vi "agent_sign.vi"() -> ()   [LabVIEW 2017]
doc: "Illustrates how to sign data using an ssh2-agent."
uses:
  libssh2/libssh2_init_default.vi
  libssh2/libssh2_session_init_ex.vi
  libssh2/libssh2.lvlib
panel:
  out "signature":string
  in  "data":string="Hello, World!"
  out "error out":errorcluster
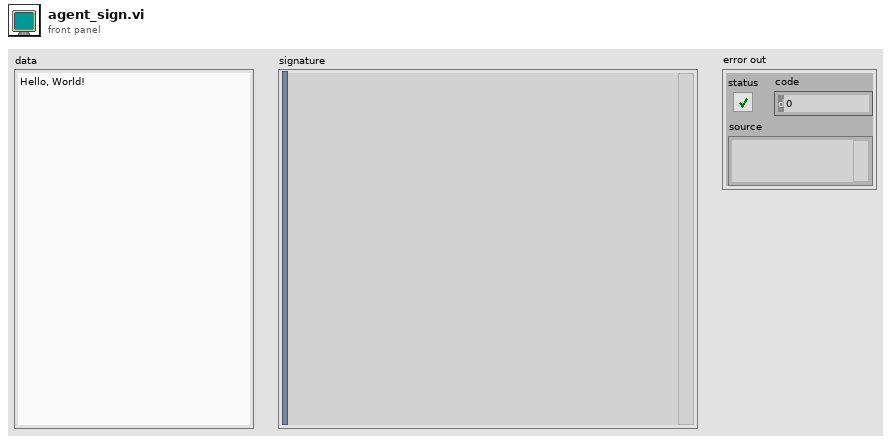
[diagram p1: front panel]
types:
  T1 = typedef "libssh2.lvlib/Session Refnum.ctl" = refnum<k1>
  T2 = typedef "libssh2.lvlib/Agent Refnum.ctl" = refnum<k1>
  T3 = typedef "libssh2.lvlib/Agent Public Key Refnum.ctl" = refnum<k1>
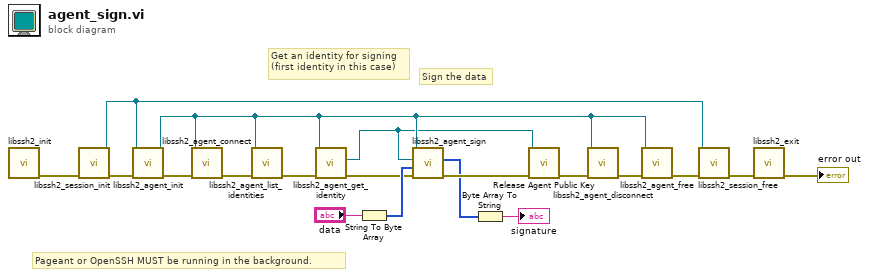
[diagram p0: block diagram]
diagram:
  # "Sign the data"
  # "Get an identity for signing\n(first identity in this case)"
  # "Pageant or OpenSSH MUST be running in the background."
  n1 = call-poly "libssh2_init.vi"() -> ("error out"=w9:errorcluster)  [unwired: 11 in]
  n2 = call "libssh2_session_init.vi"("error in (no error)"=w9) -> ("error out"=w10:errorcluster, "session"=w12:T1)  [unwired: 9 in]
  n3 = call "libssh2_agent_init.vi"("error in (no error)"=w10, "session"=w12) -> ("error out"=w16:errorcluster, "agent"=w7:T2)  [unwired: 8 in]
  n4 = call "libssh2_agent_connect.vi"("error in (no error)"=w16, "agent"=w7) -> ("error out"=w14:errorcluster)  [unwired: 9 in]
  n5 = call "libssh2_agent_list_identities.vi"("error in (no error)"=w14, "agent"=w7) -> ("error out"=w13:errorcluster)  [unwired: 9 in]
  n6 = call "libssh2_agent_get_identity.vi"("error in (no error)"=w13, "agent"=w7) -> ("error out"=w3:errorcluster, "store"=w4:T3)  [unwired: 7 in, 1 out]
  n7 = String To Byte Array(string="data") -> (unsigned byte array=w5:u8[])
  n8 = call "libssh2_agent_sign.vi"("error in (no error)"=w3, "data"=w5, "identity"=w4, "agent"=w7) -> ("error out"=w8:errorcluster, "signature"=w2:u8[])  [unwired: 6 in]
  n9 = Byte Array To String(unsigned byte array=w2) -> (string=→"signature":string)
  n10 = call "Release Agent Public Key.vi"("error in (no error)"=w8, "agent public key"=w4) -> ("error out"=w11:errorcluster)  [unwired: 9 in]
  n11 = call "libssh2_agent_disconnect.vi"("error in (no error)"=w11, "agent"=w7) -> ("error out"=w15:errorcluster)  [unwired: 9 in]
  n12 = call "libssh2_agent_free.vi"("error in (no error)"=w15, "agent"=w7) -> ("error out"=w19:errorcluster)  [unwired: 9 in]
  n13 = call "libssh2_session_free.vi"("error in (no error)"=w19, "session"=w12) -> ("error out"=w18:errorcluster)  [unwired: 9 in]
  n14 = call "libssh2_exit.vi"("error in (no error)"=w18) -> ("error out"=→"error out":errorcluster)  [unwired: 10 in]
